vi "execution class name.vi"(8 "error in":errorcluster, 11 "Calculated Tags configuration in":refnum<class "Calculated Tags configuration.lvclass">) -> (0 "error out":errorcluster, 2 "class name":string, 3 "Calculated Tags configuration out":refnum<class "Calculated Tags configuration.lvclass">)   [LabVIEW 2014, in "Calculated Tags configuration.lvclass"]
doc: "Provides an interface for determining the module runtime class associated with this module configuration. This class name can then be used to dynamically load or locate the runtime class for initialization purposes."
uses:
  Calculated Tags configuration.lvclass
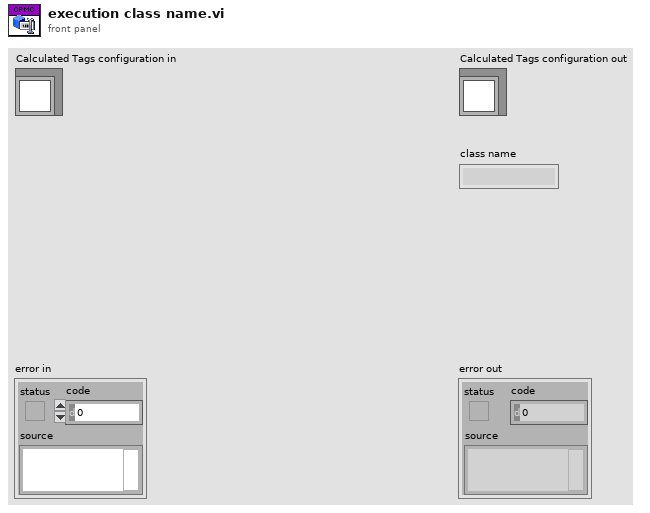
[diagram p1: front panel]
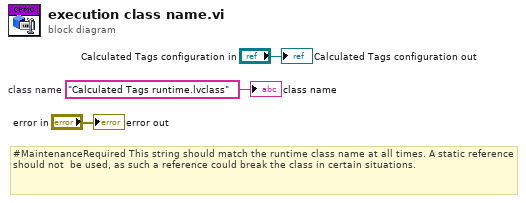
[diagram p0: block diagram]
diagram:
  w1 = "Calculated Tags runtime.lvclass"  # class name
  # "#MaintenanceRequired This string should match the runtime class name at all times. A static reference should not  be used, as such a reference could break the class in certain situations."
  "error out" <- "error in"
  "Calculated Tags configuration out" <- "Calculated Tags configuration in"
  "class name" <- w1
